vi "stepcontroller_microstepp.vi"(5 "microstep":bool, 6 "motor stopp":bool, 7 "Direction":bool) -> (0 "Boolean":bool, 1 "Boolean 2":bool, 2 "Boolean 3":bool, 3 "Boolean 4":bool)   [LabVIEW 2017]
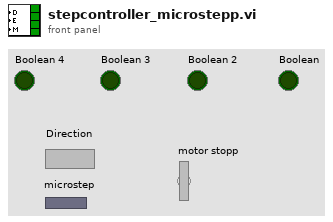
[diagram p1: front panel]
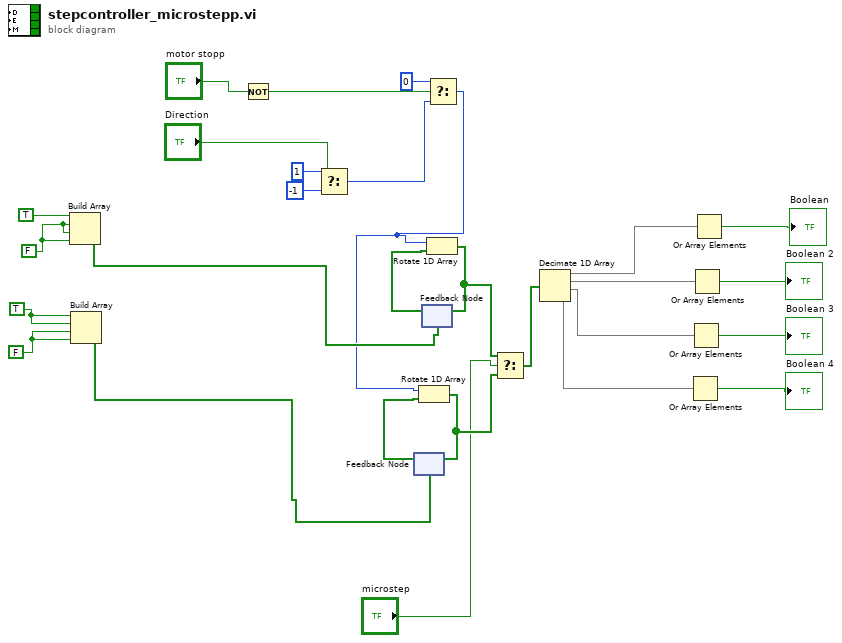
[diagram p0: block diagram]
diagram:
  w25 = FALSE
  w26 = TRUE
  w23 = FALSE
  n1 = Build Array(TRUE, w23, w23, w23) -> (w28:bool[])
  n2 = Build Array(w26, w26, w25, w25) -> (w27:bool[])
  n3 = Not(x="motor stopp") -> (.not. x?=w1:bool)
  n4 = Select(t=1, s="Direction", f=-1) -> (s? t:f=w4:i32)
  n5 = feedback #1(w27) -> (w14:bool[])
  n6 = feedback #2(w28) -> (w22:bool[])
  n7 = Select(t=0, s=w1, f=w4) -> (s? t:f=w5:i32)
  n8 = Rotate 1D Array(1:w14, 2:w5) -> (0:w12:bool[])
  n9 = feedback-in #1(w12) -> ()
  n10 = Rotate 1D Array(1:w22, 2:w5) -> (0:w13:bool[])
  n11 = feedback-in #2(w13) -> ()
  n12 = Select(t=w13, s="microstep", f=w12) -> (s? t:f=w11:bool[])
  n13 = Decimate 1D Array(w11) -> (w9:bool[], w8:bool[], w7:bool[], w6:bool[])
  n14 = Or Array Elements(Boolean array=w6) -> (logical OR=→"Boolean 4":bool)
  n15 = Or Array Elements(Boolean array=w7) -> (logical OR=→"Boolean 3":bool)
  n16 = Or Array Elements(Boolean array=w8) -> (logical OR=→"Boolean 2":bool)
  n17 = Or Array Elements(Boolean array=w9) -> (logical OR=→"Boolean":bool)
